vi "Lab Panel V5.0.vi"() -> ()   [LabVIEW 2013] (continued)
                  frame #3 {
                    n2675 = local read "on loops"() -> (w4611:dbl)
                    n2676 = local read "jig cycle"() -> (w4608:dbl)
                    n2677 = local read "Send Mail Now"() -> (w4602:bool)
                    n2678 = Add(x=w4611, y=3.0) -> (x+y=w4609:dbl)
                    n2679 = Equal?(x=w4608, y=w4609) -> (x = y?=w4603:bool)
                    n2680 = And(x=w4603, y=w4602) -> (x .and. y?=w4601:bool)
                    n2681 = And(x=w4607, y=w4603) -> (x .and. y?=w4606:bool)
                    n2682 = And(x=w4606, y=w4605) -> (x .and. y?=w4604:bool)
                    n2683 = Or(x=w4604, y=w4601) -> (x .or. y?=w4600:bool)
                    n2684 = case shown="True" w4600 {
                      tunnel: w4616 -> [_ w4622]
                      tunnel: w4615 -> [_ w4621]
                      tunnel: "Lab Panel Test Status" -> [_ w4620]
                      tunnel: w4613 -> [_ w4619]
                      tunnel: w4612 -> [_ w4618]
                      tunnel: w4599 -> [_ w4617]
                      frame False {
                      }
                      frame True {
                        n2685 = stacked-sequence {
                          tunnel: w4622 -> [w4630 _]
                          tunnel: w4621 -> [w4629 _]
                          tunnel: w4620 -> [w4628 _]
                          tunnel: w4619 -> [w4627 _]
                          tunnel: w4618 -> [w4626 _]
                          tunnel: w4617 -> [w4625 _]
                          frame #0 {
                            n2686 = call "sub vi - send mail with attach v5.vi"("TO:"=w4630, "subject"=w4628, "from"=w4626, "out going server"=w4627, "message"=w4629) -> ("error out"=w4624:errorcluster)  [unwired: 10 in]
                            n2687 = Bundle(cluster=w4625, "mail error"=w4624) -> (w4623:T6)  [unwired: 6 in]
                            n2688 = local write "MAIL SETTINGS"(w4623) -> ()
                          }
                          frame #1 {
                            n2689 = local write "mail control"("") -> ()
                            n2690 = local write "Send Mail Now"(FALSE) -> ()
                          }
                        }
                      }
                    }
                  }
                }
              }
            }
          }
          frame #18 {
            # "save jig cycle values once all run switches are off"
            n2691 = stacked-sequence {
              tunnel: w4642 -> [_ w4671]
              tunnel: w4641 -> [_ w4670]
              tunnel: w4640 -> [_ w4669]
              tunnel: w4639 -> [_ w4668]
              tunnel: w4638 -> [_ w4667]
              tunnel: w4637 -> [_ w4666]
              tunnel: w4636 -> [_ w4665]
              tunnel: w4635 -> [_ w4664]
              tunnel: w4634 -> [_ w4663]
              tunnel: w4633 -> [_ w4662]
              frame #0 {
              }
              frame #1 {
                n2692 = Not(x=w4662) -> (.not. x?=w4645:bool)
                n2693 = Not(x=w4670) -> (.not. x?=w4660:bool)
                n2694 = Not(x=w4667) -> (.not. x?=w4655:bool)
                n2695 = Not(x=w4665) -> (.not. x?=w4651:bool)
                n2696 = Not(x=w4663) -> (.not. x?=w4647:bool)
                n2697 = Not(x=w4671) -> (.not. x?=w4661:bool)
                n2698 = Not(x=w4669) -> (.not. x?=w4659:bool)
                n2699 = Not(x=w4666) -> (.not. x?=w4653:bool)
                n2700 = Not(x=w4668) -> (.not. x?=w4657:bool)
                n2701 = Not(x=w4664) -> (.not. x?=w4649:bool)
                n2702 = local read "Save JC"() -> (w4673:bool)
                n2703 = And(x=w4661, y=w4660) -> (x .and. y?=w4658:bool)
                n2704 = And(x=w4658, y=w4659) -> (x .and. y?=w4656:bool)
                n2705 = And(x=w4656, y=w4657) -> (x .and. y?=w4654:bool)
                n2706 = And(x=w4654, y=w4655) -> (x .and. y?=w4652:bool)
                n2707 = And(x=w4652, y=w4653) -> (x .and. y?=w4650:bool)
                n2708 = And(x=w4650, y=w4651) -> (x .and. y?=w4648:bool)
                n2709 = And(x=w4648, y=w4649) -> (x .and. y?=w4646:bool)
                n2710 = And(x=w4646, y=w4647) -> (x .and. y?=w4644:bool)
                n2711 = And(x=w4644, y=w4645) -> (x .and. y?=w4643:bool)
                n2712 = And(x=w4643, y=w4673) -> (x .and. y?=w4672:bool)
                n2713 = case shown="True" w4672 {
                  tunnel: w4643 -> [w4674 _]
                  frame False {
                    n2714 = case shown="False" w4674 {
                      frame False {
                        n2715 = local write "Save JC"(TRUE) -> ()
                      }
                      frame True {
                      }
                    }
                  }
                  frame True {
                    n2716 = stacked-sequence {
                      frame #0 {
                        n2717 = String To Path(string="c:\\crabtree\\Jig Cycles\\") -> (path=w4686:path)
                        n2718 = Build Path(base path=w4686, name or relative path="jigcycles.bin") -> (appended path=w4684:path)
                        n2719 = Create Folder(path (use dialog)=w4686) -> (error out=w4688:errorcluster)  [unwired: 2 in, 2 out]
                        n2720 = local read "JIG RELAY CYCLES"() -> (w4678:T7)
                        n2721 = call <vilib>:"Clear Errors.vi"("error in (no error)"=w4688) -> ()  [unwired: 6 in, 1 out]
                        n2722 = local write "Save JC"(FALSE) -> ()
                        n2723 = Open/Create/Replace File(file path (use dialog)=w4684, operation (0:open)=T19."replace or create") -> (refnum out=w4682:refnum<file>, error out=w4683:errorcluster)  [unwired: 4 in, 1 out]
                        n2724 = Write to Binary File(file (use dialog)=w4682, data=w4678, error in=w4683) -> (refnum out=w4681:refnum<file>, error out=w4680:errorcluster)  [unwired: 3 in, 1 out]
                        n2725 = Close File(refnum=w4681, error in=w4680) -> (error out=w4679:errorcluster)  [unwired: 1 out]
                        n2726 = local write "data file error"(w4679) -> ()
                      }
                      frame #1 {
                        n2727 = local read "JIG RELAY CYCLES"() -> (w4711:T7)
                        n2728 = Unbundle By Name(w4711) -> ("LAB01-1"=w4706:dbl, "LAB01-2"=w4705:dbl, "LAB02-1"=w4703:dbl, "LAB02-2"=w4702:dbl, "LAB03-1"=w4700:dbl, "LAB03-2"=w4697:dbl, "LAB04-1"=w4696:dbl, "LAB04-2"=w4694:dbl, "LAB05-1"=w4692:dbl, "LAB05-2"=w4690:dbl)
                        n2729 = stacked-sequence {
                          tunnel: w4706 -> [w4714 _ _ _ _ _ _ _ _ _]
                          tunnel: 1000000 -> [w4717 w4727 w4737 w4747 w4757 w4767 w4777 w4787 w4797 w4807]
                          tunnel: [w4715 _ _ _ _ _ _ _ _ _] -> w4709
                          tunnel: "TEST STATION HAS REACHED 1 MILLION CYCLES, REPLACE  CONTROL RELAYS" -> [w4713 w4725 w4735 w4745 w4755 w4765 w4775 w4785 w4795 w4805]
                          tunnel: [_ w4724 _ _ _ _ _ _ _ _] -> w4707
                          tunnel: w4705 -> [_ w4723 _ _ _ _ _ _ _ _]
                          tunnel: [_ _ w4734 _ _ _ _ _ _ _] -> w4704
                          tunnel: w4703 -> [_ _ w4733 _ _ _ _ _ _ _]
                          tunnel: w4702 -> [_ _ _ w4744 _ _ _ _ _ _]
                          tunnel: [_ _ _ w4743 _ _ _ _ _ _] -> w4701
                          tunnel: w4700 -> [_ _ _ _ w4754 _ _ _ _ _]
                          tunnel: [_ _ _ _ w4753 _ _ _ _ _] -> w4699
                          tunnel: [_ _ _ _ _ w4764 _ _ _ _] -> w4698
                          tunnel: w4697 -> [_ _ _ _ _ w4763 _ _ _ _]
                          tunnel: w4696 -> [_ _ _ _ _ _ w4774 _ _ _]
                          tunnel: [_ _ _ _ _ _ w4773 _ _ _] -> w4695
                          tunnel: w4694 -> [_ _ _ _ _ _ _ w4784 _ _]
                          tunnel: [_ _ _ _ _ _ _ w4783 _ _] -> w4693
                          tunnel: w4692 -> [_ _ _ _ _ _ _ _ w4794 _]
                          tunnel: [_ _ _ _ _ _ _ _ w4793 _] -> w4691
                          tunnel: w4690 -> [_ _ _ _ _ _ _ _ _ w4804]
                          tunnel: [_ _ _ _ _ _ _ _ _ w4803] -> w4689
                          frame #0 {
                            n2730 = Greater?(x=w4714, y=w4717) -> (0:w4716:bool)
                            n2731 = case shown="True" w4716 {
                              tunnel: [w4718 0] -> w4715
                              tunnel: w4714 -> [w4718 _]
                              tunnel: w4713 -> [_ w4719]
                              frame False {
                              }
                              frame True {
                                n2732 = Concatenate Strings("LA01-1 ", w4719) -> (w4722:string)
                                n2733 = One Button Dialog(message=w4722) -> ()  [unwired: 1 in, 1 out]
                              }
                            }
                          }
                          frame #1 {
                            n2734 = Greater?(x=w4723, y=w4727) -> (0:w4726:bool)
                            n2735 = case shown="True" w4726 {
                              tunnel: [w4728 0] -> w4724
                              tunnel: w4723 -> [w4728 _]
                              tunnel: w4725 -> [_ w4729]
                              frame False {
                              }
                              frame True {
                                n2736 = Concatenate Strings("LA01-2 ", w4729) -> (w4732:string)
                                n2737 = One Button Dialog(message=w4732) -> ()  [unwired: 1 in, 1 out]
                              }
                            }
                          }
                          frame #2 {
                            n2738 = Greater?(x=w4733, y=w4737) -> (0:w4736:bool)
                            n2739 = case shown="True" w4736 {
                              tunnel: [w4738 0] -> w4734
                              tunnel: w4733 -> [w4738 _]
                              tunnel: w4735 -> [_ w4739]
                              frame False {
                              }
                              frame True {
                                n2740 = Concatenate Strings("LA02-1 ", w4739) -> (w4742:string)
                                n2741 = One Button Dialog(message=w4742) -> ()  [unwired: 1 in, 1 out]
                              }
                            }
                          }
                          frame #3 {
                            n2742 = Greater?(x=w4744, y=w4747) -> (0:w4746:bool)
                            n2743 = case shown="True" w4746 {
                              tunnel: [w4748 0] -> w4743
                              tunnel: w4744 -> [w4748 _]
                              tunnel: w4745 -> [_ w4749]
                              frame False {
                              }
                              frame True {
                                n2744 = Concatenate Strings("LA02-2 ", w4749) -> (w4752:string)
                                n2745 = One Button Dialog(message=w4752) -> ()  [unwired: 1 in, 1 out]
                              }
                            }
                          }
                          frame #4 {
                            n2746 = Greater?(x=w4754, y=w4757) -> (0:w4756:bool)
                            n2747 = case shown="True" w4756 {
                              tunnel: [w4758 0] -> w4753
                              tunnel: w4754 -> [w4758 _]
                              tunnel: w4755 -> [_ w4759]
                              frame False {
                              }
                              frame True {
                                n2748 = Concatenate Strings("LA03-1 ", w4759) -> (w4762:string)
                                n2749 = One Button Dialog(message=w4762) -> ()  [unwired: 1 in, 1 out]
                              }
                            }
                          }
                          frame #5 {
                            n2750 = Greater?(x=w4763, y=w4767) -> (0:w4766:bool)
                            n2751 = case shown="True" w4766 {
                              tunnel: [w4768 0] -> w4764
                              tunnel: w4763 -> [w4768 _]
                              tunnel: w4765 -> [_ w4769]
                              frame False {
                              }
                              frame True {
                                n2752 = Concatenate Strings("LA03-2 ", w4769) -> (w4772:string)
                                n2753 = One Button Dialog(message=w4772) -> ()  [unwired: 1 in, 1 out]
                              }
                            }
                          }
                          frame #6 {
                            n2754 = Greater?(x=w4774, y=w4777) -> (0:w4776:bool)
                            n2755 = case shown="True" w4776 {
                              tunnel: [w4778 0] -> w4773
                              tunnel: w4774 -> [w4778 _]
                              tunnel: w4775 -> [_ w4779]
                              frame False {
                              }
                              frame True {
                                n2756 = Concatenate Strings("LA04-1 ", w4779) -> (w4782:string)
                                n2757 = One Button Dialog(message=w4782) -> ()  [unwired: 1 in, 1 out]
                              }
                            }
                          }
                          frame #7 {
                            n2758 = Greater?(x=w4784, y=w4787) -> (0:w4786:bool)
                            n2759 = case shown="True" w4786 {
                              tunnel: [w4788 0] -> w4783
                              tunnel: w4784 -> [w4788 _]
                              tunnel: w4785 -> [_ w4789]
                              frame False {
                              }
                              frame True {
                                n2760 = Concatenate Strings("LA04-2 ", w4789) -> (w4792:string)
                                n2761 = One Button Dialog(message=w4792) -> ()  [unwired: 1 in, 1 out]
                              }
                            }
                          }
                          frame #8 {
                            n2762 = Greater?(x=w4794, y=w4797) -> (0:w4796:bool)
                            n2763 = case shown="True" w4796 {
                              tunnel: [w4798 0] -> w4793
                              tunnel: w4794 -> [w4798 _]
                              tunnel: w4795 -> [_ w4799]
                              frame False {
                              }
                              frame True {
                                n2764 = Concatenate Strings("LA05-1 ", w4799) -> (w4802:string)
                                n2765 = One Button Dialog(message=w4802) -> ()  [unwired: 1 in, 1 out]
                              }
                            }
                          }
                          frame #9 {
                            n2766 = Greater?(x=w4804, y=w4807) -> (0:w4806:bool)
                            n2767 = case shown="True" w4806 {
                              tunnel: [w4808 0] -> w4803
                              tunnel: w4804 -> [w4808 _]
                              tunnel: w4805 -> [_ w4809]
                              frame False {
                              }
                              frame True {
                                n2768 = Concatenate Strings("LA05-2 ", w4809) -> (w4812:string)
                                n2769 = One Button Dialog(message=w4812) -> ()  [unwired: 1 in, 1 out]
                              }
                            }
                          }
                        }
                        n2770 = Bundle By Name(cluster=w4711, "LAB01-1"=w4709, "LAB01-2"=w4707, "LAB02-1"=w4704, "LAB02-2"=w4701, "LAB03-1"=w4699, "LAB03-2"=w4698, "LAB04-1"=w4695, "LAB04-2"=w4693, "LAB05-1"=w4691, "LAB05-2"=w4689) -> (w4710:T7)
                        n2771 = local write "JIG RELAY CYCLES"(w4710) -> ()
                      }
                    }
                  }
                }
              }
            }
          }
          frame #19 {
            # "get temperature values"
            n2772 = local read "simulate"() -> (w4825:bool)
            n2773 = local read "Temp Test Cal"() -> (w4822:dbl)
            n2774 = stacked-sequence {
              tunnel: w4825 -> [_ w4881 w4926 w4971 w5016 w5061]
              tunnel: T12 {"1  (A) cal"=1.0, "1 (V) cal"=1.0, "1 (PF) cal"=1.0, "1 (TL) cal"=1.0, "1 (TN) cal"=1.0, "2 (A) cal"=1.0, "2 (V) cal"=1.0, "2 (PF) cal"=1.0, "2 (TL) cal"=1.0, "2 (TN) cal"=1.0} ("CAL LAB01") -> [_ w4880 w4925 w4970 w5015 w5060]
              tunnel: w4823 -> [_ w4878 _ _ _ _]
              tunnel: w4822 -> [_ w4874 w4924 w4969 w5014 w5059]
              tunnel: w4821 -> [_ w4869 _ _ _ _]
              tunnel: w4820 -> [_ _ w4915 _ _ _]
              tunnel: w4819 -> [_ _ w4914 _ _ _]
              tunnel: w4818 -> [_ _ _ w4960 _ _]
              tunnel: w4817 -> [_ _ _ w4959 _ _]
              tunnel: w4816 -> [_ _ _ _ w5005 _]
              tunnel: w4815 -> [_ _ _ _ w5004 _]
              tunnel: w4814 -> [_ _ _ _ _ w5050]
              tunnel: w4813 -> [_ _ _ _ _ w5049]
              frame #0 {
                n2775 = local read "Select COM port"() -> (w4830:refnum<visa-resource-name>)
                "COM port" <- w4830
                n2776 = local read "jig cycle"() -> (w4831:dbl)
                n2777 = local read "on loops"() -> (w4833:dbl)
                n2778 = global write "Global 1.vi" "tmp dly lps"("Temp Delay Lps") -> ()
                n2779 = global write "Global 1.vi" "dly value"("Temp Value") -> ()
                n2780 = Add(x=w4833, y=3) -> (x+y=w4834:dbl)
                n2781 = global write "Global 1.vi" "COM port"(w4830) -> ()
                n2782 = Equal?(x=w4831, y=w4834) -> (x = y?=w4827:bool)
                n2783 = local read "Temp Loops"() -> (w4826:dbl)
                n2784 = case shown="True" w4827 {
                  tunnel: w4826 -> [_ w4836]
                  frame False {
                  }
                  frame True {
                    n2785 = stacked-sequence {
                      tunnel: w4836 -> [w4839 w4867]
                      frame #0 {
                        n2786 = local read "simulate"() -> (w4837:bool)
                        n2787 = case shown="5" w4839 {
                          tunnel: 1.0 -> [_ w4844 w4846 w4852 w4856 w4861]
                          tunnel: w4837 -> [_ w4840 w4845 w4850 w4857 w4860]
                          frame 0, Default {
                          }
                          frame 1 {
                            w4842 = FALSE
                            n2788 = call "sub vi - GET ALL TEMP v5.vi"("LA01-EN"=TRUE, "simulate"=w4840, "LA02-EN"=w4842, "LA03-EN"=w4842, "LA04-EN"=w4842, "LA05-EN"=w4842, "Gen Cal Value"=w4844) -> ("LA01 TEMP"=w4841:T22)  [unwired: 3 in, 5 out]
                            n2789 = local write "LAB01 TEMP"(w4841) -> ()
                          }
                          frame 2 {
                            w4847 = FALSE
                            n2790 = call "sub vi - GET ALL TEMP v5.vi"("LA01-EN"=w4847, "simulate"=w4845, "LA02-EN"=TRUE, "LA03-EN"=w4847, "LA04-EN"=w4847, "LA05-EN"=w4847, "Gen Cal Value"=w4846) -> ("LA02 TEMP"=w4849:T22)  [unwired: 3 in, 5 out]
                            n2791 = local write "LAB02 TEMP"(w4849) -> ()
                          }
                          frame 3 {
                            w4853 = FALSE
                            n2792 = call "sub vi - GET ALL TEMP v5.vi"("LA01-EN"=w4853, "simulate"=w4850, "LA02-EN"=w4853, "LA03-EN"=TRUE, "LA04-EN"=w4853, "LA05-EN"=w4853, "Gen Cal Value"=w4852) -> ("LA03 TEMP"=w4851:T22)  [unwired: 3 in, 5 out]
                            n2793 = local write "LAB03 TEMP"(w4851) -> ()
                          }
                          frame 4 {
                            w4858 = FALSE
                            n2794 = call "sub vi - GET ALL TEMP v5.vi"("LA01-EN"=w4858, "simulate"=w4857, "LA02-EN"=w4858, "LA03-EN"=w4858, "LA04-EN"=TRUE, "LA05-EN"=w4858, "Gen Cal Value"=w4856) -> ("LA04 TEMP"=w4855:T22)  [unwired: 3 in, 5 out]
                            n2795 = local write "LAB04 TEMP"(w4855) -> ()
                          }
                          frame 5 {
                            w4863 = FALSE
                            n2796 = call "sub vi - GET ALL TEMP v5.vi"("LA01-EN"=w4863, "simulate"=w4860, "LA02-EN"=w4863, "LA03-EN"=w4863, "LA04-EN"=w4863, "LA05-EN"=TRUE, "Gen Cal Value"=w4861) -> ("LA05 TEMP"=w4862:T22)  [unwired: 3 in, 5 out]
                            n2797 = local write "LAB05 TEMP"(w4862) -> ()
                          }
                        }
                      }
                      frame #1 {
                        n2798 = Greater Or Equal?(x=w4867, y=5) -> (x >= y?=w4865:bool)
                        n2799 = case shown="True" w4865 {
                          frame False {
                          }
                          frame True {
                            n2800 = local write "Temp Loops"(0) -> ()
                          }
                        }
                      }
                    }
                    n2801 = local write "TEMP"(TRUE) -> ()
                  }
                }
              }
              frame #1 {
                n2802 = case shown="False" w4881 {
                  tunnel: [w4912 w4913] -> w4897
                  tunnel: w4880 -> [_ w4913]
                  frame False {
                    n2803 = local read "CAL LAB01"() -> (w4912:T12)
                  }
                  frame True {
                  }
                }
                n2804 = local read "LAB01 TEMP"() -> (w4887:T11)
                n2805 = local read "TEMP LA01"() -> (w4888:T8)
                n2806 = call "sub vi - temperature delay v2.vi"("temp values IN"=w4888, "temp signals"=w4887) -> ("T2-N"=w4883:dbl, "T2-L"=w4884:dbl, "T1-N"=w4885:dbl, "T1-L"=w4886:dbl, "temp values OUT"=w4882:T39)  [unwired: 5 in]
                n2807 = Unbundle By Name(w4897) -> ("1 (TL) cal"=w4892:dbl, "1 (TN) cal"=w4891:dbl, "2 (TL) cal"=w4890:dbl, "2 (TN) cal"=w4889:dbl)  [unwired: 6 out]
                n2808 = local write "TEMP LA01"(w4882) -> ()
                n2809 = Multiply(x=w4886, y=w4892) -> (x*y=w4879:dbl)
                n2810 = Multiply(x=w4885, y=w4891) -> (x*y=w4876:dbl)
                n2811 = Multiply(x=w4884, y=w4890) -> (x*y=w4873:dbl)
                n2812 = Multiply(x=w4883, y=w4889) -> (x*y=w4872:dbl)
                n2813 = case shown="True" w4878 {
                  tunnel: w4879 -> [w4906 w4911]
                  tunnel: w4874 -> [_ w4909]
                  tunnel: [w4906 w4910] -> w4877
                  tunnel: w4876 -> [w4905 w4908]
                  tunnel: [w4905 w4907] -> w4875
                  frame False {
                  }
                  frame True {
                    n2814 = Multiply(x=w4909, y=w4908) -> (x*y=w4907:dbl)
                    n2815 = Multiply(x=w4909, y=w4911) -> (x*y=w4910:dbl)
                  }
                }
                n2816 = case shown="True" w4869 {
                  tunnel: w4873 -> [w4899 w4904]
                  tunnel: w4874 -> [_ w4902]
                  tunnel: [w4899 w4903] -> w4871
                  tunnel: w4872 -> [w4898 w4901]
                  tunnel: [w4898 w4900] -> w4870
                  frame False {
                  }
                  frame True {
                    n2817 = Multiply(x=w4902, y=w4901) -> (x*y=w4900:dbl)
                    n2818 = Multiply(x=w4902, y=w4904) -> (x*y=w4903:dbl)
                  }
                }
                n2819 = local read "SIG LAB01-2"() -> (w4894:T2)
                n2820 = local read "SIG LAB01-1"() -> (w4896:T2)
                n2821 = Bundle By Name(cluster=w4896, "Tmp Live"=w4877, "Tmp Neut"=w4875) -> (w4895:T2)
                n2822 = Bundle By Name(cluster=w4894, "Tmp Live"=w4871, "Tmp Neut"=w4870) -> (w4893:T2)
                n2823 = local write "SIG LAB01-1"(w4895) -> ()
                n2824 = local write "SIG LAB01-2"(w4893) -> ()
              }
              frame #2 {
                n2825 = case shown="True" w4926 {
                  tunnel: [w4957 w4958] -> w4942
                  tunnel: w4925 -> [_ w4958]
                  frame False {
                    n2826 = local read "CAL LAB02"() -> (w4957:T13)
                  }
                  frame True {
                  }
                }
                n2827 = local read "LAB02 TEMP"() -> (w4933:T11)
                n2828 = local read "TEMP LA02"() -> (w4932:T8)
                n2829 = call "sub vi - temperature delay v2.vi"("temp values IN"=w4932, "temp signals"=w4933) -> ("T2-N"=w4927:dbl, "T2-L"=w4928:dbl, "T1-N"=w4929:dbl, "T1-L"=w4930:dbl, "temp values OUT"=w4931:T39)  [unwired: 5 in]
                n2830 = Unbundle By Name(w4942) -> ("1 (TL) cal"=w4937:dbl, "1 (TN) cal"=w4936:dbl, "2 (TL) cal"=w4935:dbl, "2 (TN) cal"=w4934:dbl)  [unwired: 6 out]
                n2831 = local write "TEMP LA02"(w4931) -> ()
                n2832 = Multiply(x=w4930, y=w4937) -> (x*y=w4923:dbl)
                n2833 = Multiply(x=w4929, y=w4936) -> (x*y=w4922:dbl)
                n2834 = Multiply(x=w4928, y=w4935) -> (x*y=w4919:dbl)
                n2835 = Multiply(x=w4927, y=w4934) -> (x*y=w4918:dbl)
                n2836 = case shown="True" w4915 {
                  tunnel: w4923 -> [w4951 w4956]
                  tunnel: w4924 -> [_ w4954]
                  tunnel: [w4951 w4955] -> w4921
                  tunnel: w4922 -> [w4950 w4953]
                  tunnel: [w4950 w4952] -> w4920
                  frame False {
                  }
                  frame True {
                    n2837 = Multiply(x=w4954, y=w4953) -> (x*y=w4952:dbl)
                    n2838 = Multiply(x=w4954, y=w4956) -> (x*y=w4955:dbl)
                  }
                }
                n2839 = case shown="True" w4914 {
                  tunnel: w4919 -> [w4944 w4949]
                  tunnel: w4924 -> [_ w4947]
                  tunnel: [w4944 w4948] -> w4917
                  tunnel: w4918 -> [w4943 w4946]
                  tunnel: [w4943 w4945] -> w4916
                  frame False {
                  }
                  frame True {
                    n2840 = Multiply(x=w4947, y=w4946) -> (x*y=w4945:dbl)
                    n2841 = Multiply(x=w4947, y=w4949) -> (x*y=w4948:dbl)
                  }
                }
                n2842 = local read "SIG LAB02-2"() -> (w4939:T2)
                n2843 = local read "SIG LAB02-1"() -> (w4941:T2)
                n2844 = Bundle By Name(cluster=w4941, "Tmp Live"=w4921, "Tmp Neut"=w4920) -> (w4940:T2)
                n2845 = Bundle By Name(cluster=w4939, "Tmp Live"=w4917, "Tmp Neut"=w4916) -> (w4938:T2)
                n2846 = local write "SIG LAB02-1"(w4940) -> ()
                n2847 = local write "SIG LAB02-2"(w4938) -> ()
              }
              frame #3 {
                n2848 = case shown="False" w4971 {
                  tunnel: [w5002 w5003] -> w4987
                  tunnel: w4970 -> [_ w5003]
                  frame False {
                    n2849 = local read "CAL LAB03"() -> (w5002:T12)
                  }
                  frame True {
                  }
                }
                n2850 = local read "TEMP LA03"() -> (w4977:T8)
                n2851 = local read "LAB03 TEMP"() -> (w4978:T11)
                n2852 = call "sub vi - temperature delay v2.vi"("temp values IN"=w4977, "temp signals"=w4978) -> ("T2-N"=w4972:dbl, "T2-L"=w4973:dbl, "T1-N"=w4974:dbl, "T1-L"=w4975:dbl, "temp values OUT"=w4976:T39)  [unwired: 5 in]
                n2853 = Unbundle By Name(w4987) -> ("1 (TL) cal"=w4982:dbl, "1 (TN) cal"=w4981:dbl, "2 (TL) cal"=w4980:dbl, "2 (TN) cal"=w4979:dbl)  [unwired: 6 out]
                n2854 = local write "TEMP LA03"(w4976) -> ()
                n2855 = Multiply(x=w4975, y=w4982) -> (x*y=w4968:dbl)
                n2856 = Multiply(x=w4974, y=w4981) -> (x*y=w4967:dbl)
                n2857 = Multiply(x=w4973, y=w4980) -> (x*y=w4964:dbl)
                n2858 = Multiply(x=w4972, y=w4979) -> (x*y=w4963:dbl)
                n2859 = case shown="True" w4959 {
                  tunnel: w4964 -> [w4989 w4994]
                  tunnel: w4969 -> [_ w4992]
                  tunnel: [w4989 w4993] -> w4962
                  tunnel: w4963 -> [w4988 w4991]
                  tunnel: [w4988 w4990] -> w4961
                  frame False {
                  }
                  frame True {
                    n2860 = Multiply(x=w4992, y=w4991) -> (x*y=w4990:dbl)
                    n2861 = Multiply(x=w4992, y=w4994) -> (x*y=w4993:dbl)
                  }
                }
                n2862 = case shown="True" w4960 {
                  tunnel: w4968 -> [w4996 w5001]
                  tunnel: w4969 -> [_ w4999]
                  tunnel: [w4996 w5000] -> w4966
                  tunnel: w4967 -> [w4995 w4998]
                  tunnel: [w4995 w4997] -> w4965
                  frame False {
                  }
                  frame True {
                    n2863 = Multiply(x=w4999, y=w4998) -> (x*y=w4997:dbl)
                    n2864 = Multiply(x=w4999, y=w5001) -> (x*y=w5000:dbl)
                  }
                }
                n2865 = local read "SIG LAB03-2"() -> (w4984:T2)
                n2866 = local read "SIG LAB03-1"() -> (w4986:T2)
                n2867 = Bundle By Name(cluster=w4986, "Tmp Live"=w4966, "Tmp Neut"=w4965) -> (w4985:T2)
                n2868 = Bundle By Name(cluster=w4984, "Tmp Live"=w4962, "Tmp Neut"=w4961) -> (w4983:T2)
                n2869 = local write "SIG LAB03-1"(w4985) -> ()
                n2870 = local write "SIG LAB03-2"(w4983) -> ()
              }
              frame #4 {
                n2871 = case shown="False" w5016 {
                  tunnel: [w5047 w5048] -> w5032
                  tunnel: w5015 -> [_ w5048]
                  frame False {
                    n2872 = local read "CAL LAB04"() -> (w5047:T12)
                  }
                  frame True {
                  }
                }
                n2873 = local read "LAB04 TEMP"() -> (w5022:T11)
                n2874 = local read "TEMP LA04"() -> (w5023:T8)
                n2875 = call "sub vi - temperature delay v2.vi"("temp values IN"=w5023, "temp signals"=w5022) -> ("T2-N"=w5017:dbl, "T2-L"=w5018:dbl, "T1-N"=w5019:dbl, "T1-L"=w5020:dbl, "temp values OUT"=w5021:T39)  [unwired: 5 in]
                n2876 = Unbundle By Name(w5032) -> ("1 (TL) cal"=w5027:dbl, "1 (TN) cal"=w5026:dbl, "2 (TL) cal"=w5025:dbl, "2 (TN) cal"=w5024:dbl)  [unwired: 6 out]
                n2877 = local write "TEMP LA04"(w5021) -> ()
                n2878 = Multiply(x=w5020, y=w5027) -> (x*y=w5013:dbl)
                n2879 = Multiply(x=w5019, y=w5026) -> (x*y=w5012:dbl)
                n2880 = Multiply(x=w5018, y=w5025) -> (x*y=w5009:dbl)
                n2881 = Multiply(x=w5017, y=w5024) -> (x*y=w5008:dbl)
                n2882 = case shown="True" w5004 {
                  tunnel: w5009 -> [w5034 w5039]
                  tunnel: w5014 -> [_ w5037]
                  tunnel: [w5034 w5038] -> w5007
                  tunnel: w5008 -> [w5033 w5036]
                  tunnel: [w5033 w5035] -> w5006
                  frame False {
                  }
                  frame True {
                    n2883 = Multiply(x=w5037, y=w5036) -> (x*y=w5035:dbl)
                    n2884 = Multiply(x=w5037, y=w5039) -> (x*y=w5038:dbl)
                  }
                }
                n2885 = case shown="True" w5005 {
                  tunnel: w5013 -> [w5041 w5046]
                  tunnel: w5014 -> [_ w5044]
                  tunnel: [w5041 w5045] -> w5011
                  tunnel: w5012 -> [w5040 w5043]
                  tunnel: [w5040 w5042] -> w5010
                  frame False {
                  }
                  frame True {
                    n2886 = Multiply(x=w5044, y=w5043) -> (x*y=w5042:dbl)
                    n2887 = Multiply(x=w5044, y=w5046) -> (x*y=w5045:dbl)
                  }
                }
                n2888 = local read "SIG LAB04-2"() -> (w5029:T2)
                n2889 = local read "SIG LAB04-1"() -> (w5031:T2)
                n2890 = Bundle By Name(cluster=w5031, "Tmp Live"=w5011, "Tmp Neut"=w5010) -> (w5030:T2)
                n2891 = Bundle By Name(cluster=w5029, "Tmp Live"=w5007, "Tmp Neut"=w5006) -> (w5028:T2)
                n2892 = local write "SIG LAB04-1"(w5030) -> ()
                n2893 = local write "SIG LAB04-2"(w5028) -> ()
              }
              frame #5 {
                n2894 = case shown="False" w5061 {
                  tunnel: [w5092 w5093] -> w5077
                  tunnel: w5060 -> [_ w5093]
                  frame False {
                    n2895 = local read "CAL LAB05"() -> (w5092:T12)
                  }
                  frame True {
                  }
                }
                n2896 = local read "LAB05 TEMP"() -> (w5067:T11)
                n2897 = local read "TEMP LA05"() -> (w5068:T8)
                n2898 = call "sub vi - temperature delay v2.vi"("temp values IN"=w5068, "temp signals"=w5067) -> ("T2-N"=w5063:dbl, "T2-L"=w5064:dbl, "T1-N"=w5065:dbl, "T1-L"=w5066:dbl, "temp values OUT"=w5062:T39)  [unwired: 5 in]
                n2899 = local write "TEMP LA05"(w5062) -> ()
                n2900 = Unbundle By Name(w5077) -> ("1 (TL) cal"=w5069:dbl, "1 (TN) cal"=w5072:dbl, "2 (TL) cal"=w5071:dbl, "2 (TN) cal"=w5070:dbl)  [unwired: 6 out]
                n2901 = Multiply(x=w5066, y=w5069) -> (x*y=w5058:dbl)
                n2902 = Multiply(x=w5065, y=w5072) -> (x*y=w5057:dbl)
                n2903 = Multiply(x=w5064, y=w5071) -> (x*y=w5054:dbl)
                n2904 = Multiply(x=w5063, y=w5070) -> (x*y=w5053:dbl)
                n2905 = case shown="True" w5049 {
                  tunnel: w5054 -> [w5079 w5084]
                  tunnel: w5059 -> [_ w5082]
                  tunnel: [w5079 w5083] -> w5052
                  tunnel: w5053 -> [w5078 w5081]
                  tunnel: [w5078 w5080] -> w5051
                  frame False {
                  }
                  frame True {
                    n2906 = Multiply(x=w5082, y=w5081) -> (x*y=w5080:dbl)
                    n2907 = Multiply(x=w5082, y=w5084) -> (x*y=w5083:dbl)
                  }
                }
                n2908 = case shown="True" w5050 {
                  tunnel: w5058 -> [w5086 w5091]
                  tunnel: w5059 -> [_ w5089]
                  tunnel: [w5086 w5090] -> w5056
                  tunnel: w5057 -> [w5085 w5088]
                  tunnel: [w5085 w5087] -> w5055
                  frame False {
                  }
                  frame True {
                    n2909 = Multiply(x=w5089, y=w5088) -> (x*y=w5087:dbl)
                    n2910 = Multiply(x=w5089, y=w5091) -> (x*y=w5090:dbl)
                  }
                }
                n2911 = local read "SIG LAB05-1"() -> (w5076:T2)
                n2912 = Bundle By Name(cluster=w5076, "Tmp Live"=w5056, "Tmp Neut"=w5055) -> (w5075:T2)
                n2913 = local read "SIG LAB05-2"() -> (w5074:T2)
                n2914 = Bundle By Name(cluster=w5074, "Tmp Live"=w5052, "Tmp Neut"=w5051) -> (w5073:T2)
                n2915 = local write "SIG LAB05-1"(w5075) -> ()
                n2916 = local write "SIG LAB05-2"(w5073) -> ()
              }
            }
          }
          frame #20 {
            # "write data to display panel"
            n2917 = global write "Global display 1.vi" "TEST 5-2"(w5108) -> ()
            n2918 = global write "Global display 1.vi" "TEST 4-2"(w5110) -> ()
            n2919 = global write "Global display 1.vi" "TEST 1-2"(w5116) -> ()
            n2920 = global write "Global display 1.vi" "TEST 3-1"(w5113) -> ()
            n2921 = global write "Global display 1.vi" "TEST 5-1"(w5109) -> ()
            n2922 = global write "Global display 1.vi" "TEST 1-1"(w5117) -> ()
            n2923 = global write "Global display 1.vi" "TEST 3-2"(w5112) -> ()
            n2924 = global write "Global display 1.vi" "TEST 4-1"(w5111) -> ()
            n2925 = global write "Global display 1.vi" "TEST 2-2"(w5114) -> ()
            n2926 = global write "Global display 1.vi" "TEST 2-1"(w5115) -> ()
            n2927 = global read "Global display 3.vi" "log 1-1"() -> (→"LOG LAB01-1":string)
            n2928 = global read "Global display 3.vi" "log 3-1"() -> (→"LOG LAB03-1":string)
            n2929 = global read "Global display 3.vi" "log 1-2"() -> (→"LOG LAB01-2":string)
            n2930 = property on="Tab Control 2" class="TabCtl (strict)"() -> ("Pages"=w5107:refnum<vi>[])  [unwired: 2 in, 2 out]
            n2931 = global read "Global display 3.vi" "log 2-1"() -> (→"LOG LAB02-1":string)
            n2932 = global read "Global display 3.vi" "log 2-2"() -> (→"LOG LAB02-2":string)
            n2933 = global read "Global display 3.vi" "log 4-2"() -> (→"LOG LAB04-2":string)
            n2934 = global read "Global display 3.vi" "log 5-2"() -> (→"LOG LAB05-2":string)
            n2935 = global read "Global display 3.vi" "log 5-1"() -> (→"LOG LAB05-1":string)
            n2936 = global read "Global display 3.vi" "log 4-1"() -> (→"LOG LAB04-1":string)
            n2937 = global read "Global display 3.vi" "log 3-2"() -> (→"LOG LAB03-2":string)
            n2938 = Index Array(array=w5107, index=9) -> (element=w5105:refnum<vi>)
            n2939 = property class="Page"(reference=w5105) -> ("PageVis"=w5104:bool)  [unwired: 1 in, 2 out]
            n2940 = global write "Global display 3.vi" "admin"(w5104) -> ()
            n2941 = local read "O/I  LAB05-2"() -> (w5158:bool)
            n2942 = local read "O/I  LAB05-1"() -> (w5159:bool)
            n2943 = local read "O/I  LAB03-2"() -> (w5162:bool)
            n2944 = local read "O/I  LAB04-2"() -> (w5160:bool)
            n2945 = local read "O/I  LAB04-1"() -> (w5161:bool)
            n2946 = local read "O/I  LAB03-1"() -> (w5163:bool)
            n2947 = local read "O/I  LAB01-2"() -> (w5166:bool)
            n2948 = local read "O/I  LAB01-1"() -> (w5167:bool)
            n2949 = local read "O/I  LAB02-1"() -> (w5165:bool)
            n2950 = local read "O/I  LAB02-2"() -> (w5164:bool)
            n2951 = global write "Global display 1.vi" "5-2 O/F"(w5158) -> ()
            n2952 = global write "Global display 1.vi" "5-1 O/F"(w5159) -> ()
            n2953 = global write "Global display 1.vi" "4-1 O/F"(w5161) -> ()
            n2954 = global write "Global display 1.vi" "4-2 O/F"(w5160) -> ()
            n2955 = global write "Global display 1.vi" "3-2 O/F"(w5162) -> ()
            n2956 = global write "Global display 1.vi" "3-1 O/F"(w5163) -> ()
            n2957 = global write "Global display 1.vi" "2-2 O/F"(w5164) -> ()
            n2958 = global write "Global display 1.vi" "2-1 O/F"(w5165) -> ()
            n2959 = global write "Global display 1.vi" "1-2 O/F"(w5166) -> ()
            n2960 = global write "Global display 1.vi" "1-1 O/F"(w5167) -> ()
            n2961 = local read "run lab05-2"() -> (w5148:bool)
            n2962 = local read "run lab04-1"() -> (w5151:bool)
            n2963 = local read "run lab04-2"() -> (w5150:bool)
            n2964 = local read "run lab05-1"() -> (w5149:bool)
            n2965 = local read "run lab03-2"() -> (w5152:bool)
            n2966 = local read "run lab02-1"() -> (w5155:bool)
            n2967 = local read "run lab03-1"() -> (w5153:bool)
            n2968 = local read "run lab01-2"() -> (w5156:bool)
            n2969 = local read "run lab02-2"() -> (w5154:bool)
            n2970 = local read "run lab01-1"() -> (w5157:bool)
            n2971 = global write "Global display 1.vi" "5-2 R/S"(w5148) -> ()
            n2972 = global write "Global display 1.vi" "5-1 R/S"(w5149) -> ()
            n2973 = global write "Global display 1.vi" "4-2 R/S"(w5150) -> ()
            n2974 = global write "Global display 1.vi" "4-1 R/S"(w5151) -> ()
            n2975 = global write "Global display 1.vi" "3-2 R/S"(w5152) -> ()
            n2976 = global write "Global display 1.vi" "1-2 R/S"(w5156) -> ()
            n2977 = global write "Global display 1.vi" "2-1 R/S"(w5155) -> ()
            n2978 = global write "Global display 1.vi" "3-1 R/S"(w5153) -> ()
            n2979 = global write "Global display 1.vi" "2-2 R/S"(w5154) -> ()
            n2980 = global write "Global display 1.vi" "1-1 R/S"(w5157) -> ()
            n2981 = local read "DISP LAB04-2"() -> (w5140:T4)
            n2982 = local read "DISP LAB05-1"() -> (w5139:T4)
            n2983 = local read "DISP LAB04-1"() -> (w5141:T4)
            n2984 = local read "DISP LAB05-2"() -> (w5138:T4)
            n2985 = local read "DISP LAB03-1"() -> (w5143:T4)
            n2986 = local read "DISP LAB03-2"() -> (w5142:T4)
            n2987 = local read "DISP LAB01-2"() -> (w5146:T4)
            n2988 = local read "DISP LAB02-1"() -> (w5145:T4)
            n2989 = local read "DISP LAB02-2"() -> (w5144:T4)
            n2990 = local read "DISP LAB01-1"() -> (w5147:T4)
            n2991 = global write "Global display 2.vi" "DISP LAB05-1"(w5139) -> ()
            n2992 = global write "Global display 2.vi" "DISP LAB05-2"(w5138) -> ()
            n2993 = global write "Global display 2.vi" "DISP LAB04-2"(w5140) -> ()
            n2994 = global write "Global display 2.vi" "DISP LAB02-1"(w5145) -> ()
            n2995 = global write "Global display 2.vi" "DISP LAB02-2"(w5144) -> ()
            n2996 = global write "Global display 2.vi" "DISP LAB04-1"(w5141) -> ()
            n2997 = global write "Global display 2.vi" "DISP LAB01-2"(w5146) -> ()
            n2998 = global write "Global display 2.vi" "DISP LAB01-1"(w5147) -> ()
            n2999 = global write "Global display 2.vi" "DISP LAB03-1"(w5143) -> ()
            n3000 = global write "Global display 2.vi" "DISP LAB03-2"(w5142) -> ()
            n3001 = local read "SET LAB05-2"() -> (w5128:T5)
            n3002 = local read "SET LAB05-1"() -> (w5129:T5)
            n3003 = local read "SET LAB04-1"() -> (w5131:T5)
            n3004 = local read "SET LAB04-2"() -> (w5130:T5)
            n3005 = local read "SET LAB03-1"() -> (w5133:T5)
            n3006 = local read "SET LAB03-2"() -> (w5132:T5)
            n3007 = local read "SET LAB02-2"() -> (w5134:T5)
            n3008 = local read "SET LAB01-2"() -> (w5136:T5)
            n3009 = local read "SET LAB02-1"() -> (w5135:T5)
            n3010 = local read "SET LAB01-1"() -> (w5137:T5)
            n3011 = global write "Global display 2.vi" "SET LAB05-2"(w5128) -> ()
            n3012 = global write "Global display 2.vi" "SET LAB05-1"(w5129) -> ()
            n3013 = global write "Global display 2.vi" "SET LAB04-1"(w5131) -> ()
            n3014 = global write "Global display 2.vi" "SET LAB04-2"(w5130) -> ()
            n3015 = global write "Global display 2.vi" "SET LAB03-2"(w5132) -> ()
            n3016 = global write "Global display 2.vi" "SET LAB02-2"(w5134) -> ()
            n3017 = global write "Global display 2.vi" "SET LAB03-1"(w5133) -> ()
            n3018 = global write "Global display 2.vi" "SET LAB01-2"(w5136) -> ()
            n3019 = global write "Global display 2.vi" "SET LAB01-1"(w5137) -> ()
            n3020 = global write "Global display 2.vi" "SET LAB02-1"(w5135) -> ()
            n3021 = local read "RESULT LAB01-1"() -> (w5127:bool)
            n3022 = local read "RESULT LAB03-2"() -> (w5122:bool)
            n3023 = local read "RESULT LAB04-1"() -> (w5121:bool)
            n3024 = local read "RESULT LAB04-2"() -> (w5120:bool)
            n3025 = local read "RESULT LAB02-2"() -> (w5124:bool)
            n3026 = local read "RESULT LAB01-2"() -> (w5126:bool)
            n3027 = local read "RESULT LAB02-1"() -> (w5125:bool)
            n3028 = local read "RESULT LAB03-1"() -> (w5123:bool)
            n3029 = local read "RESULT LAB05-1"() -> (w5119:bool)
            n3030 = local read "RESULT LAB05-2"() -> (w5118:bool)
            n3031 = global write "Global display 2.vi" "RESULT LAB05-1"(w5119) -> ()
            n3032 = global write "Global display 2.vi" "RESULT LAB01-2"(w5126) -> ()
            n3033 = global write "Global display 2.vi" "RESULT LAB03-2"(w5122) -> ()
            n3034 = global write "Global display 2.vi" "RESULT LAB04-1"(w5121) -> ()
            n3035 = global write "Global display 2.vi" "RESULT LAB04-2"(w5120) -> ()
            n3036 = global write "Global display 2.vi" "RESULT LAB05-2"(w5118) -> ()
            n3037 = global write "Global display 2.vi" "RESULT LAB03-1"(w5123) -> ()
            n3038 = global write "Global display 2.vi" "RESULT LAB02-1"(w5125) -> ()
            n3039 = global write "Global display 2.vi" "RESULT LAB02-2"(w5124) -> ()
            n3040 = global write "Global display 2.vi" "RESULT LAB01-1"(w5127) -> ()
          }
          frame #21 {
            # "end main and display program"
            n3041 = Quit LabVIEW(quit? (T)="stop all") -> ()
            n3042 = event shown="[1] \"CALIBRATION\": Value Change" {
              selector: _ -> [_ _]
              dyn-events: _ -> [_ _]
              timeout: 10 -> [_ _]
              event Timeout {
                n3043 = event-data() -> ()  [unwired: 1 in, 3 out]
              }
              event "CALIBRATION": Value Change {
                n3044 = event-data() -> ()  [unwired: 1 in, 6 out]
              }
            }
            n3045 = global write "Global display 1.vi" "stop disp"("stop all") -> ()
          }
        }
        n3046 = node-c288() -> ()  [unwired: 1 in, 1 out]
        "loops" <- w287
      }
      n3047 = node-c288(w264) -> ()  [unwired: 1 out]
    }
  }
